vi "BlinkM GoToRGB.vi"(0 "Arduino Resource":T1={"VISA resource"="", "Board Type"=enum."Uno", "Connection Type"=enum."USB / Serial", "Bytes Per Packet (15)"=15}, 5 "Address (0)":u8, 9 "Color":u32(colorbox), 11 "error in":errorcluster) -> (4 "Arduino Resource":T1={"VISA resource"="", "Board Type"=enum."Uno", "Connection Type"=enum."USB / Serial", "Bytes Per Packet (15)"=15}, 15 "error out":errorcluster)   [LabVIEW 2015, in "LabVIEW Interface for Arduino.lvlib"]
doc: "Set the BlinkM to the specified RGB color immediatly."
uses:
  <vilib>/LabVIEW Interface for Arduino/LabVIEW Interface for Arduino.lvlib
  <vilib>/LabVIEW Interface for Arduino/Type Defs/Arduino Resource.ctl
  <vilib>/LabVIEW Interface for Arduino/Type Defs/Board Type.ctl
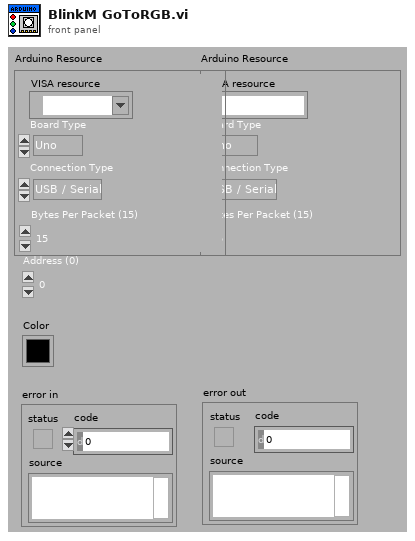
[diagram p1: front panel]
types:
  T1 = typedef "LabVIEW Interface for Arduino.lvlib/Arduino Resource.ctl" = cluster{"VISA resource":refnum<visa-resource-name>, "Board Type":T2, "Connection Type":enum8{"USB / Serial"}, "Bytes Per Packet (15)":u8}
  T2 = typedef "LabVIEW Interface for Arduino.lvlib/Board Type.ctl" = enum16{"Uno", "Dimuelanove w/Atmega 328", "Mega 2560"}
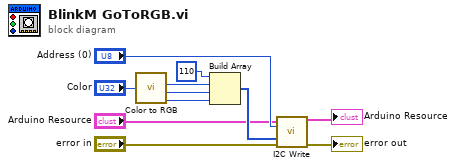
[diagram p0: block diagram]
diagram:
  n1 = call <vilib>:"Color to RGB.vi"("Color"="Color") -> ("R"=w7:u8, "G"=w6:u8, "B"=w5:u8)  [unwired: 1 out]
  n2 = Build Array(u8 110 ("new element/subarray"), w7, w6, w5) -> (w3:u8[])
  n3 = call <vilib>:"I2C Write.vi"("Arduino Resource"="Arduino Resource", "Address (0)"="Address (0)", "I2C Data Bytes"=w3, "error in"="error in") -> ("Arduino Resource"=→"Arduino Resource":T1, "error out"=→"error out":errorcluster)  [unwired: 10 in]
